vi "VectorCased.vi"(11 "XYUVArray":dbl[][](array[numeric])=[[-138.0, 28.0, -5.0, -3.0], [-92.0, 28.0, -10.0, -5.5], [-46.0, 28.0, -5.0, -10.5], [0.0, 28.0, -9.0, 3.5], [46.0, 28.0, -22.0, 1.0], [92.0, 28.0, -24.5, -9.0], [138.0, 28.0, -16.0, -23.0], [-138.0, 60.0, -6.0, -2.0], [-92.0, 60.0, -7.0, -12.0], [-46.0, 60.0, -6.0, -11.0], [0.0, 60.0, -9.0, 3.0], [46.0, 60.0, -5.5, 6.0], [92.0, 60.0, -10.0, -7.5], [138.0, 60.0, -17.0, -22.0], [-138.0, 92.0, 0.5, 2.0], [-92.0, 92.0, -1.5, -15.0], [-46.0, 92.0, -1.5, -10.5], [0.0, 92.0, 1.0, -1.5], [46.0, 92.0, 1.0, 3.0], [92.0, 92.0, -2.5, -7.5], [138.0, 92.0, -5.0, -17.0], [-138.0, 124.0, 18.5, 15.0], [-92.0, 124.0, 10.5, -2.5], [-46.0, 124.0, 6.5, -2.0], [0.0, 124.0, 7.5, 5.0], [46.0, 124.0, 9.5, 12.5], [92.0, 124.0, 14.0, 8.5], [138.0, 124.0, 6.5, -4.0], [-138.0, 156.0, 13.5, 14.5], [-92.0, 156.0, 19.5, 4.0], [-46.0, 156.0, 12.5, -1.0], [0.0, 156.0, 10.5, 3.5], [46.0, 156.0, 14.0, 11.0], [92.0, 156.0, 17.5, 10.5], [138.0, 156.0, 12.0, -4.5], [-138.0, 188.0, 9.0, 16.5], [-92.0, 188.0, 10.0, 8.0], [-46.0, 188.0, 14.0, 4.0], [0.0, 188.0, 15.5, 8.0], [46.0, 188.0, 14.5, 11.0], [92.0, 188.0, 21.5, 11.0], [138.0, 188.0, 19.0, 0.5], [-138.0, 214.0, 12.5, 11.5], [-92.0, 214.0, 17.5, 6.0], [-46.0, 214.0, 17.0, 9.5], [0.0, 214.0, 14.5, 10.5], [46.0, 214.0, 19.0, 10.5], [92.0, 214.0, 20.0, 7.0], [138.0, 214.0, 16.5, 7.0]]) -> ()   [LabVIEW 2011]
panel:
  in  "ArrowScale":dbl(slide)=0.3 min=0.0 step=0.1 scale=0.0..0.5
  in  "stop":bool
  in  "Border":dbl(slide)=0.2 min=0.0 step=0.05 scale=0.0..0.2
  in  "VectorScale":dbl(slide)=1.5 min=0.0 step=0.25 scale=0.0..100.0
  out "VectorPicture":picture
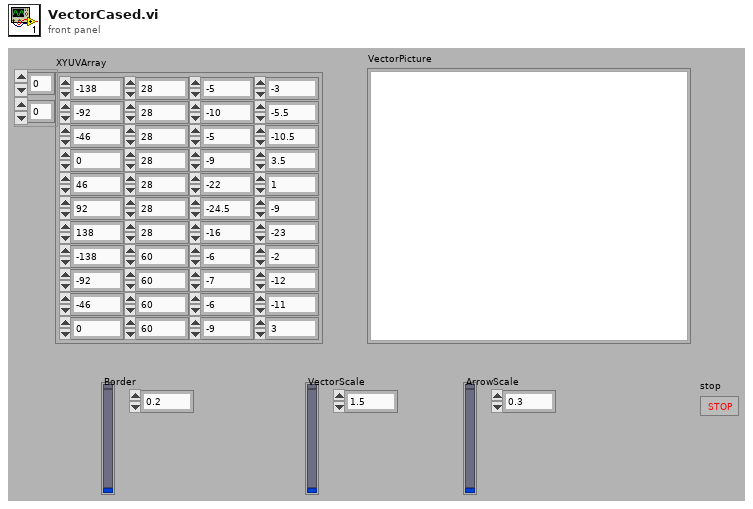
[diagram p1: front panel]
types:
  T1 = typedef "LVBoundsTypeDef.ctl" = cluster{"Width":u32, "Height":u32}
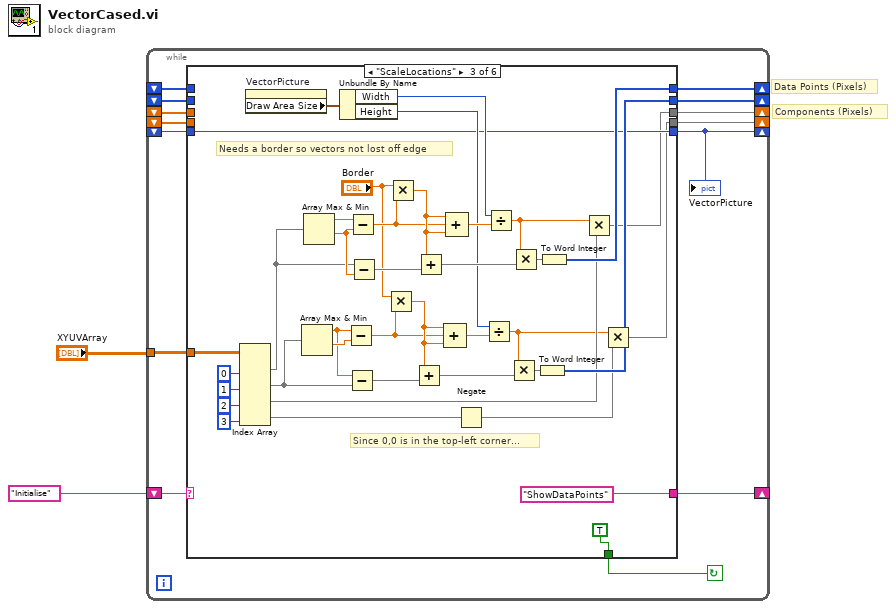
[diagram p0: block diagram]
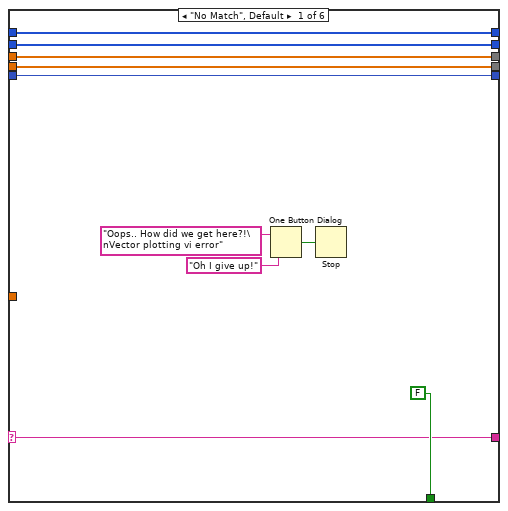
[diagram p2: hidden frame]
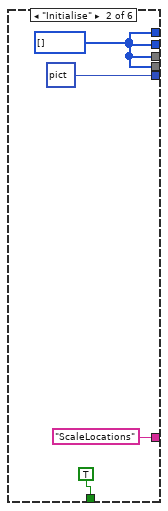
[diagram p3: hidden frame]
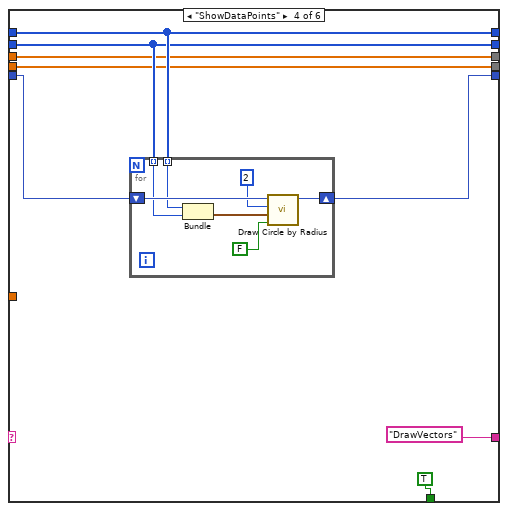
[diagram p4: hidden frame]
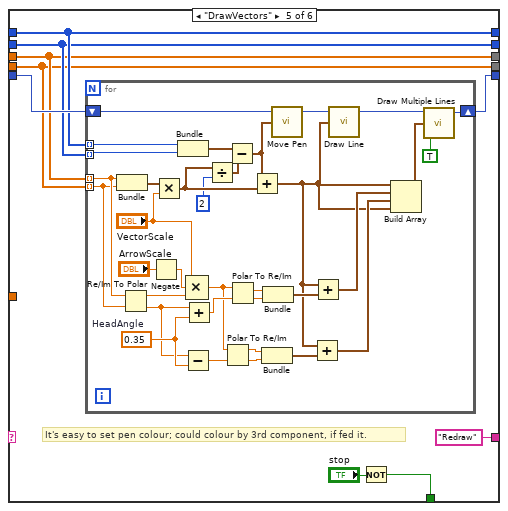
[diagram p5: hidden frame]
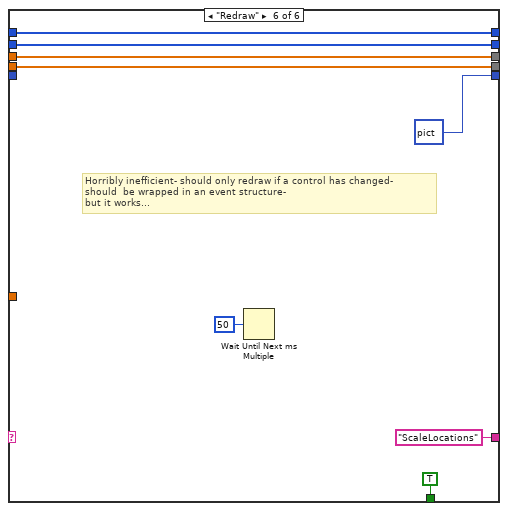
[diagram p6: hidden frame]
diagram:
  # "Components (Pixels)"
  # "Data Points (Pixels)"
  n1 = while {
    shift-right: [w12] -> _
    shift-left: "Initialise" -> [w16]
    shift-right: [w7] -> _
    shift-left: _ -> [w14]
    shift-right: [w11] -> _
    shift-left: _ -> [w9]
    shift-right: [w10] -> _
    shift-left: _ -> [w8]
    shift-right: [w6] -> _
    shift-left: _ -> [w4]
    shift-right: [w5] -> _
    shift-left: _ -> [w3]
    tunnel: "XYUVArray" -> [w13]
    stop <- w15 continue-if-true
    n2 = case shown="\"ScaleLocations\"" w16 {
      selector: w16 -> [w25 _ _ _ _ _]
      tunnel: [FALSE TRUE TRUE TRUE w85 TRUE] -> w15
      tunnel: [w24 picture data[5B] ("new picture") w34 w73 w92 picture data[5B] ("new picture")] -> w7
      tunnel: w14 -> [w24 _ w34 w77 w93 _]
      tunnel: w13 -> [_ _ w31 _ _ _]
      tunnel: [w25 "ScaleLocations" "ShowDataPoints" "DrawVectors" "Redraw" "ScaleLocations"] -> w12
      tunnel: [w23 w27 w44 w76 w91 w135] -> w11
      tunnel: [w22 w27 w43 w75 w90 w134] -> w10
      tunnel: w9 -> [w23 _ _ w76 w91 w135]
      tunnel: w8 -> [w22 _ _ w75 w90 w134]
      tunnel: [w21 w27 w33 w72 w89 w133] -> w6
      tunnel: [w20 w27 w32 w71 w88 w132] -> w5
      tunnel: w4 -> [w21 _ _ w72 w89 w133]
      tunnel: w3 -> [w20 _ _ w71 w88 w132]
      frame "No Match", Default {
        n3 = One Button Dialog(message="Oops.. How did we get here?!\nVector plotting vi error", button name ("OK")="Oh I give up!") -> (true=w17:bool)
        n4 = Stop(stop? (T)=w17) -> ()
      }
      frame "Initialise" {
        w27 = i16[] []
      }
      frame "ScaleLocations" {
        # "Needs a border so vectors not lost off edge"
        # "Since 0,0 is in the top-left corner..."
        n5 = Index Array(array=w31, index (col) #1=0 ("disabled index (col)"), index (col) #2=1 ("index (col)"), index (col) #3=2 ("index (col)"), index (col) #4=3 ("index (col)")) -> (element #1=w63:dbl[], element #2=w49:dbl[], element #3=w39:dbl[], element #4=w36:dbl[])  [unwired: 4 in]
        n6 = property on="VectorPicture" class="Pict"() -> ("Draw Area Size"=w42:T1)  [unwired: 2 in, 2 out]
        n7 = Array Max & Min(array=w49) -> (max value=w50:dbl, min value=w54:dbl)  [unwired: 2 out]
        n8 = Array Max & Min(array=w63) -> (max value=w69:dbl, min value=w64:dbl)  [unwired: 2 out]
        n9 = Unbundle By Name(w42) -> ("Width"=w41:u32, "Height"=w40:u32)
        n10 = Subtract(x=w50, y=w54) -> (x-y=w51:dbl)
        n11 = Subtract(x=w50, y=w49) -> (x-y=w55:dbl[])
        n12 = Subtract(x=w69, y=w64) -> (x-y=w53:dbl)
        n13 = Subtract(x=w63, y=w64) -> (x-y=w62:dbl[])
        n14 = Multiply(x="Border", y=w51) -> (x*y=w56:dbl)
        n15 = Multiply(x="Border", y=w53) -> (x*y=w61:dbl)
        n16 = Add(x=w56, y=w55) -> (x+y=w58:dbl[])
        n17 = Add(x=w61, y=w62) -> (x+y=w59:dbl[])
        n18 = Compound Arithmetic op=ADD(w56, w51, w56) -> (w57:dbl)
        n19 = Compound Arithmetic op=ADD(w61, w53, w61) -> (w60:dbl)
        n20 = Negate(x=w36) -> (-x=w35:dbl[])
        n21 = Divide(x=w40, y=w57) -> (x/y=w37:dbl)
        n22 = Divide(x=w41, y=w60) -> (x/y=w38:dbl)
        n23 = Multiply(x=w37, y=w58) -> (x*y=w45:dbl[])
        n24 = Multiply(x=w38, y=w59) -> (x*y=w46:dbl[])
        n25 = To Word Integer(number=w45) -> (16bit integer=w43:i16[])
        n26 = To Word Integer(number=w46) -> (16bit integer=w44:i16[])
        n27 = Multiply(x=w38, y=w39) -> (x*y=w33:dbl[])
        n28 = Multiply(x=w37, y=w35) -> (x*y=w32:dbl[])
      }
      frame "ShowDataPoints" {
        n29 = for {
          tunnel: w76 -> [w79] mode=indexing
          tunnel: w75 -> [w78] mode=indexing
          shift-right: [w84] -> w73
          shift-left: w77 -> [w82]
          n30 = Bundle(w79, w78) -> (w80:cluster{i16, i16})  [unwired: 1 in]
          n31 = call <vilib>:"Draw Circle by Radius.vi"("fill?(F)"=FALSE, "pixel center"=w80, "radius"=i16 2, "picture"=w82) -> ("new picture"=w84:picture)  [unwired: 7 in]
        }
      }
      frame "DrawVectors" {
        # "It's easy to set pen colour; could colour by 3rd component, if fed it."
        n32 = for {
          tunnel: w89 -> [w117] mode=indexing
          tunnel: w88 -> [w116] mode=indexing
          tunnel: w91 -> [w126] mode=indexing
          tunnel: w90 -> [w125] mode=indexing
          shift-right: [w119] -> w92
          shift-left: w93 -> [w127]
          w105 = 0.35  # HeadAngle
          n33 = Bundle(w117, w116) -> (w120:cluster{dbl, dbl})  [unwired: 1 in]
          n34 = Re/Im To Polar(2:w116, 3:w117) -> (0:w104:dbl, 1:w111:dbl)
          n35 = Negate(x="ArrowScale") -> (-x=w95:dbl)
          n36 = Multiply(x=w120, y="VectorScale") -> (x*y=w124:cluster{dbl, dbl})
          n37 = Bundle(w126, w125) -> (w122:cluster{i16, i16})  [unwired: 1 in]
          n38 = Subtract(x=w104, y=w105) -> (x-y=w101:dbl)
          n39 = Add(x=w104, y=w105) -> (x+y=w112:dbl)
          n40 = Compound Arithmetic op=MULTIPLY("VectorScale", w95, w111) -> (w100:dbl)
          n41 = Divide(x=w124, y=2) -> (x/y=w121:cluster{dbl, dbl})
          n42 = Polar To Re/Im(2:w101, 3:w100) -> (0:w103:dbl, 1:w102:dbl)
          n43 = Subtract(x=w122, y=w121) -> (x-y=w109:cluster{dbl, dbl})
          n44 = Polar To Re/Im(2:w112, 3:w100) -> (0:w114:dbl, 1:w115:dbl)
          n45 = Add(x=w109, y=w124) -> (x+y=w96:cluster{dbl, dbl})
          n46 = Bundle(w102, w103) -> (w99:cluster{dbl, dbl})  [unwired: 1 in]
          n47 = Bundle(w115, w114) -> (w113:cluster{dbl, dbl})  [unwired: 1 in]
          n48 = call <vilib>:"Move Pen.vi"("new position"=w109, "picture"=w127) -> ("new picture"=w107:picture)  [unwired: 3 in]
          n49 = Add(x=w96, y=w99) -> (x+y=w97:cluster{dbl, dbl})
          n50 = Add(x=w96, y=w113) -> (x+y=w98:cluster{dbl, dbl})
          n51 = call <vilib>:"Draw Line.vi"("picture"=w107, "end point"=w96) -> ("new picture"=w106:picture)  [unwired: 7 in]
          n52 = Build Array(w96, w98, w97, w96) -> (w118:cluster{dbl, dbl}[])
          n53 = call <vilib>:"Draw Multiple Lines.vi"("picture"=w106, "line endpoints"=w118, "fill?(F)"=TRUE) -> ("new picture"=w119:picture)  [unwired: 6 in]
        }
        n54 = Not(x="stop") -> (.not. x?=w85:bool)
      }
      frame "Redraw" {
        # "Horribly inefficient- should only redraw if a control has changed-\nshould  be wrapped in an event structure-\nbut it works..."
        n55 = Wait Until Next ms Multiple(millisecond multiple=u32 50) -> ()  [unwired: 1 out]
      }
    }
    "VectorPicture" <- w7
  }
